vi "streamingDataWriter.vi"() -> ()   [LabVIEW 2012]
uses:
  <userlib>/Common/Communication/ActiveMQ/ActiveMQBroker/ActiveMQBroker.lvclass
panel:
  out "Waveform Chart":dbl[](graph)
  in  "stopWriter":bool
  in  "topic":string="testTopic"
  in  "port":string="61616"
  in  "host":string="localhost"
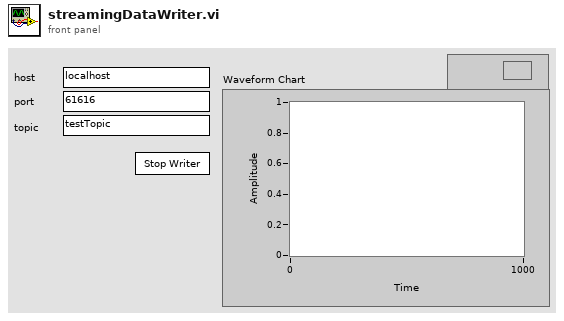
[diagram p1: front panel]
types:
  T1 = enum32{"invalid app kind", "Development System", "Run Time System", "Student Edition", "Embedded LabVIEW", "Evaluation", "Custom"}
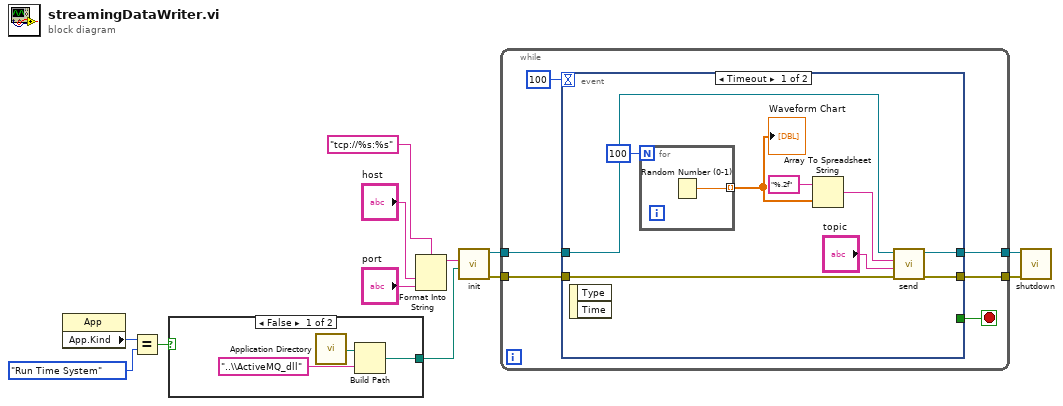
[diagram p0: block diagram]
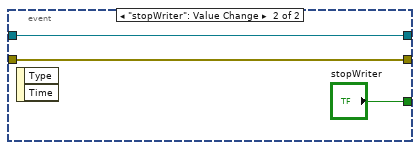
[diagram p2: hidden frame]
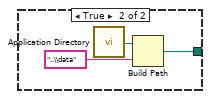
[diagram p3: hidden frame]
diagram:
  n1 = property class="App"() -> ("App.Kind"=w9:T1)  [unwired: 2 in, 2 out]
  n2 = Equal?(x=w9, y=T1."Run Time System") -> (x = y?=w7:bool)
  n3 = case shown="False" w7 {
    tunnel: [w13 w16] -> w12
    frame False {
      n4 = call <vilib>:"Application Directory.vi"() -> ("Application Directory"=w14:path)
      n5 = Build Path(base path=w14, name or relative path="..\\ActiveMQ_dll") -> (appended path=w13:path)
    }
    frame True {
      n6 = call <vilib>:"Application Directory.vi"() -> ("Application Directory"=w18:path)
      n7 = Build Path(base path=w18, name or relative path="..\\data") -> (appended path=w16:path)
    }
  }
  n8 = Format Into String(format string="tcp://%s:%s", "host", "port") -> (resulting string=w5:string)  [unwired: 2 in, 1 out]
  n9 = call <userlib>:"init.vi"("activeMQ_dll_directory"=w12, "brokerConnectionString"=w5) -> ("error out"=w1:errorcluster, "ActiveMQBroker out"=w2:refnum<class "ActiveMQBroker.lvclass">)  [unwired: 7 in, 1 out]
  n10 = while {
    tunnel: [w24] -> w11
    tunnel: [w23] -> w10
    tunnel: w2 -> [w22]
    tunnel: w1 -> [w21]
    stop <- w20 stop-if-true
    n11 = event shown="[0] Timeout" {
      selector: _ -> [_ _]
      dyn-events: _ -> [_ _]
      timeout: 100 -> [_ _]
      tunnel: [w33 w36] -> w24
      tunnel: [w32 w35] -> w23
      tunnel: w22 -> [w30 w36]
      tunnel: w21 -> [w29 w35]
      tunnel: [_ "stopWriter"] -> w20
      event Timeout {
        n12 = event-data() -> ()  [unwired: 1 in, 2 out]
        n13 = for {
          N: 100 -> [_]
          tunnel: [w34] -> w26 mode=indexing
          n14 = Random Number (0-1)() -> (number: 0 to 1=w34:dbl)
        }
        "Waveform Chart" <- w26
        n15 = Array To Spreadsheet String(array=w26, 3:"%.2f" ("format string")) -> (spreadsheet string=w28:string)  [unwired: 1 in]
        n16 = call-dynamic "send.vi"("error in (no error)"=w29, "topic"="topic", "message"=w28, "ActiveMQBroker in"=w30) -> ("error out"=w32:errorcluster, "ActiveMQBroker out"=w33:refnum<class "ActiveMQBroker.lvclass">)  [unwired: 6 in]
      }
      event "stopWriter": Value Change {
        n17 = event-data() -> ()  [unwired: 1 in, 2 out]
      }
    }
  }
  n18 = call-dynamic "shutdown.vi"("error in (no error)"=w10, "ActiveMQBroker in"=w11) -> ()  [unwired: 8 in, 2 out]
